vi "温度报警.vi"() -> ()   [LabVIEW 2022 SP3]
panel:
  in  "报警上限":dbl(slide) scale=0.0..100.0
  in  "停止":bool
  out "报警灯":bool
  in  "报警开关":bool
  out "温度计":dbl(slide) scale=0.0..100.0
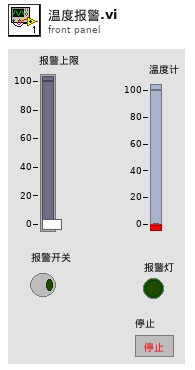
[diagram p1: front panel]
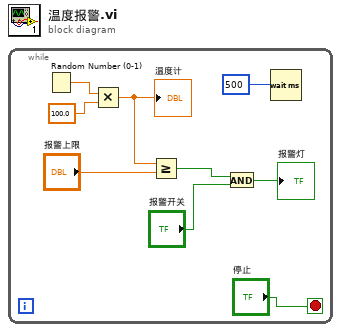
[diagram p0: block diagram]
diagram:
  n1 = while {
    stop <- "停止" stop-if-true
    n2 = Random Number (0-1)() -> (number: 0 to 1=w9:dbl)
    n3 = Multiply(x=w9, y=100.0) -> (x*y=w7:dbl)
    "温度计" <- w7
    n4 = Greater Or Equal?(x=w7, y="报警上限") -> (x >= y?=w5:bool)
    n5 = And(x=w5, y="报警开关") -> (x .and. y?=→"报警灯":bool)
    n6 = Wait (ms)(milliseconds to wait=500) -> ()  [unwired: 1 out]
  }
